vi "GetPressedButton.vi"(9 "Present Mode":u8, 10 "Cluster":refnum<vi>, 11 "Array in":refnum<vi>) -> (0 "Valid":bool, 1 "Button Changed?":bool, 2 "Parameter":string, 3 "Index":u32, 5 "Phase Name":string)   [LabVIEW 2018, in "Visualization.lvlib" / "VisualizeAcPwr.lvclass"]
uses:
  AcPwr/VisualizeAcPwr.lvclass
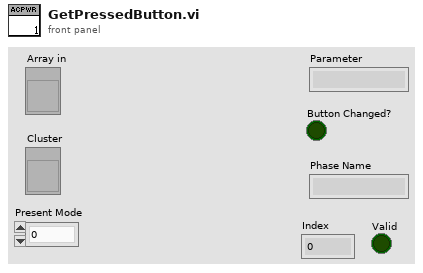
[diagram p1: front panel]
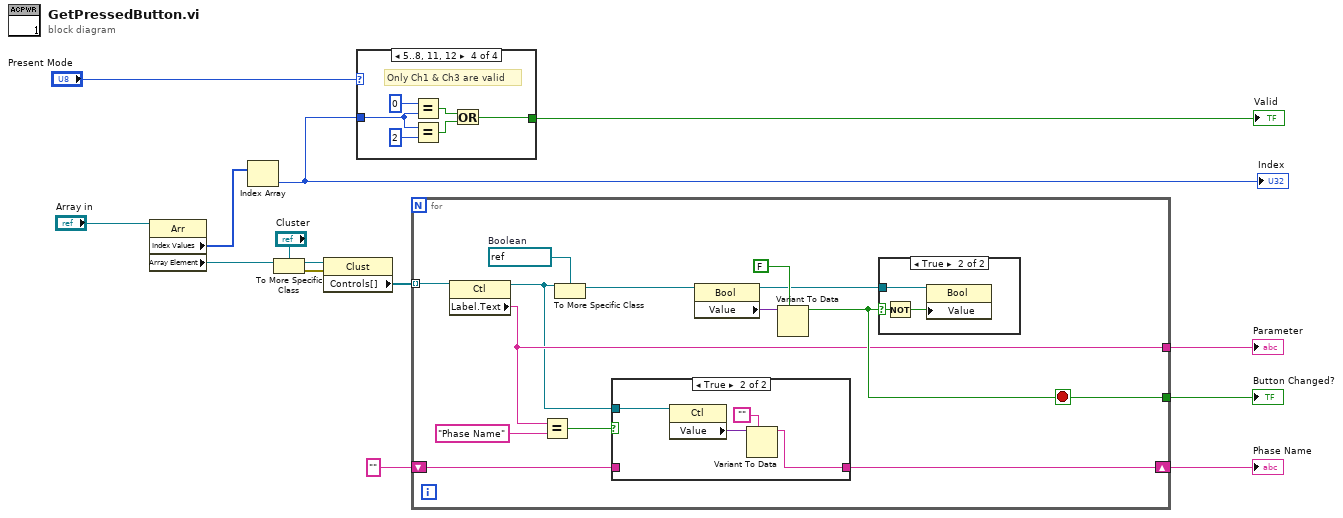
[diagram p0: block diagram]
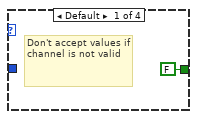
[diagram p4: hidden frame]
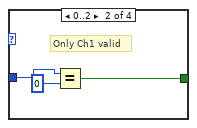
[diagram p5: hidden frame]
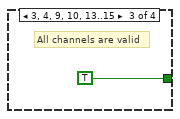
[diagram p6: hidden frame]
diagram:
  n1 = property class="Arr"(reference="Array in") -> ("Index Values"=w10:u32[], "Array Element"=w14:refnum<vi>)  [unwired: 1 in, 2 out]
  n2 = Index Array(array=w10) -> (element=w7:u32)  [unwired: 1 in]
  "Index" <- w7
  n3 = To More Specific Class(target class="Cluster", reference=w14) -> (specific class reference=w3:refnum<vi>, error out=w4:errorcluster)  [unwired: 1 in]
  n4 = property class="Clust"(reference=w3, error in=w4) -> ("Controls[]"=w5:refnum<vi>[])  [unwired: 2 out]
  n5 = case shown="5..8, 11, 12" "Present Mode" {
    tunnel: w7 -> [_ w18 _ w22]
    tunnel: [FALSE w16 TRUE w23] -> w6
    frame Default {
      # "Don't accept values if channel is not valid"
    }
    frame 0..2 {
      # "Only Ch1 valid"
      n6 = Equal?(x=w18, y=u32 0) -> (x = y?=w16:bool)
    }
    frame 3, 4, 9, 10, 13..15 {
      # "All channels are valid"
    }
    frame 5..8, 11, 12 {
      # "Only Ch1 & Ch3 are valid"
      n7 = Equal?(x=u32 0, y=w22) -> (x = y?=w25:bool)
      n8 = Equal?(x=w22, y=u32 2) -> (x = y?=w24:bool)
      n9 = Or(x=w25, y=w24) -> (x .or. y?=w23:bool)
    }
  }
  "Valid" <- w6
  n10 = for {
    tunnel: w5 -> [w38] mode=indexing
    tunnel: [w31] -> w12
    tunnel: [w32] -> w11
    shift-right: [w28] -> w9
    shift-left: "" ("y") -> [w27]
    stop <- w32 stop-if-true
    w37 = refnum<vi> refnum  # Boolean
    n11 = property class="Ctl"(reference=w38) -> (reference out=w26:refnum<vi>, "Label.Text"=w31:string)  [unwired: 1 in, 1 out]
    n12 = Equal?(x=w31, y="Phase Name") -> (x = y?=w30:bool)
    n13 = To More Specific Class(target class=w37, reference=w26) -> (specific class reference=w36:refnum<vi>)  [unwired: 1 in, 1 out]
    n14 = case shown="True" w30 {
      tunnel: [w39 w40] -> w28
      tunnel: w27 -> [w39 _]
      tunnel: w26 -> [_ w43]
      frame False {
      }
      frame True {
        n15 = property class="Ctl"(reference=w43) -> ("Value"=w42:variant)  [unwired: 1 in, 2 out]
        n16 = Variant To Data(type="", Variant=w42) -> (data=w40:string)  [unwired: 1 in, 1 out]
      }
    }
    n17 = property class="Bool"(reference=w36) -> (reference out=w33:refnum<vi>, "Value"=w35:variant)  [unwired: 1 in, 1 out]
    n18 = Variant To Data(type=FALSE, Variant=w35) -> (data=w32:bool)  [unwired: 1 in, 1 out]
    n19 = case shown="True" w32 {
      selector: w32 -> [_ w45]
      tunnel: w33 -> [_ w46]
      frame False {
      }
      frame True {
        n20 = Not(x=w45) -> (.not. x?=w44:bool)
        n21 = property class="Bool"(reference=w46, "Value"=w44) -> ()  [unwired: 1 in, 2 out]
      }
    }
  }
  "Parameter" <- w12
  "Button Changed?" <- w11
  "Phase Name" <- w9
